vi "Generate Blend Points.vi"(6 "Index":i32, 8 "Speeds":T2={"maxV (fps)"=20.0, "Accel Limit (fps^2)"=20.0, "Initial V (fps)"=0.0, "Sample Period (s)"=0.02, "Jerk Limit (fps^3)"=0.0, "Jerk Distances"={"distance (ft)"=0.0, 0.0, 0.0}, "Jerk Distances"={"distance (ft)"=0.0, 0.0, 0.0}}, 9 "Initial Point":cluster{"x":dbl, "y":dbl, "th":dbl}={"x"=1.0, "y"=2.0, "th"=30.0}, 10 "Initial Acceleration":dbl format="%#_13g", 11 "Blend Info":T1) -> (0 "Speeds Out":T2={"maxV (fps)"=20.0, "Accel Limit (fps^2)"=20.0, "Initial V (fps)"=0.0, "Sample Period (s)"=0.02, "Jerk Limit (fps^3)"=0.0, "Jerk Distances"={"distance (ft)"=0.0, 0.0, 0.0}, "Jerk Distances"={"distance (ft)"=0.0, 0.0, 0.0}}, 3 "Trajectory Segment":T3, 5 "Final Acceleration":dbl)   [LabVIEW 2019]
uses:
  BlendType.ctl
panel:
  out "XY Graph":cluster{cluster{dbl, dbl}[]}[](graph)
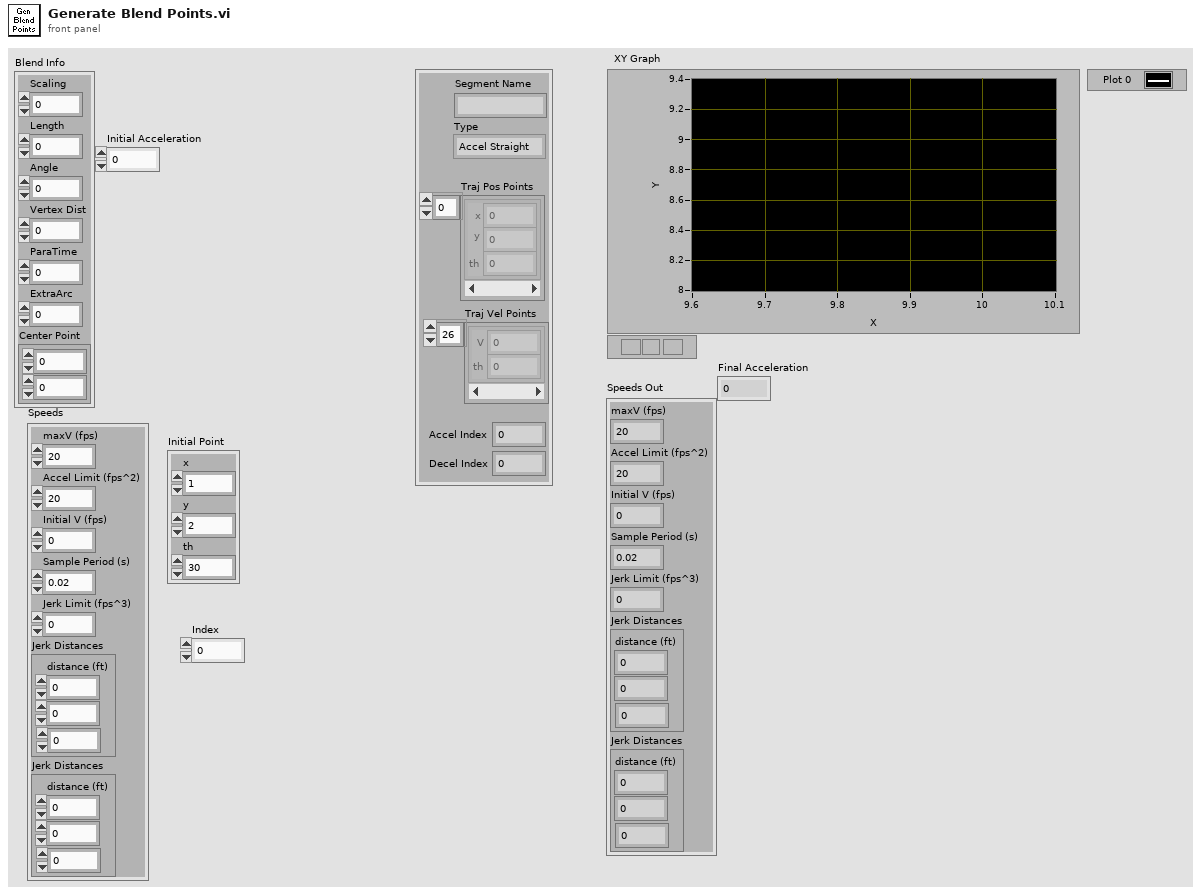
[diagram p1: front panel]
types:
  T1 = typedef "BlendType.ctl" = cluster{"Scaling":dbl, "Length":dbl, "Angle":dbl, "Vertex Dist":dbl, "ParaTime":dbl, "ExtraArc":dbl, "Center Point":cluster{dbl, dbl}}
  T2 = cluster{"maxV (fps)":dbl, "Accel Limit (fps^2)":dbl, "Initial V (fps)":dbl, "Sample Period (s)":dbl, "Jerk Limit (fps^3)":dbl, "Jerk Distances":cluster{"distance (ft)":dbl, dbl, dbl}, "Jerk Distances":cluster{"distance (ft)":dbl, dbl, dbl}}
  T3 = cluster{"Segment Name":string, "Type":enum16{"Accel Straight", "Const Straight", "Blend", "Circle"}, "Traj Pos Points":cluster{"x":dbl, "y":dbl, "th":dbl}[], "Traj Vel Points":cluster{"V":dbl, "th":dbl}[], "Accel Index":i32, "Decel Index":i32}
  T4 = enum16{"Accel Straight", "Const Straight", "Blend", "Circle"}
  T5 = cluster{string, "Type":enum16{"Accel Straight", "Const Straight", "Blend", "Circle"}, cluster{dbl, dbl, dbl}[], cluster{dbl, dbl}[], "Accel Index":i32, "Decel Index":i32}
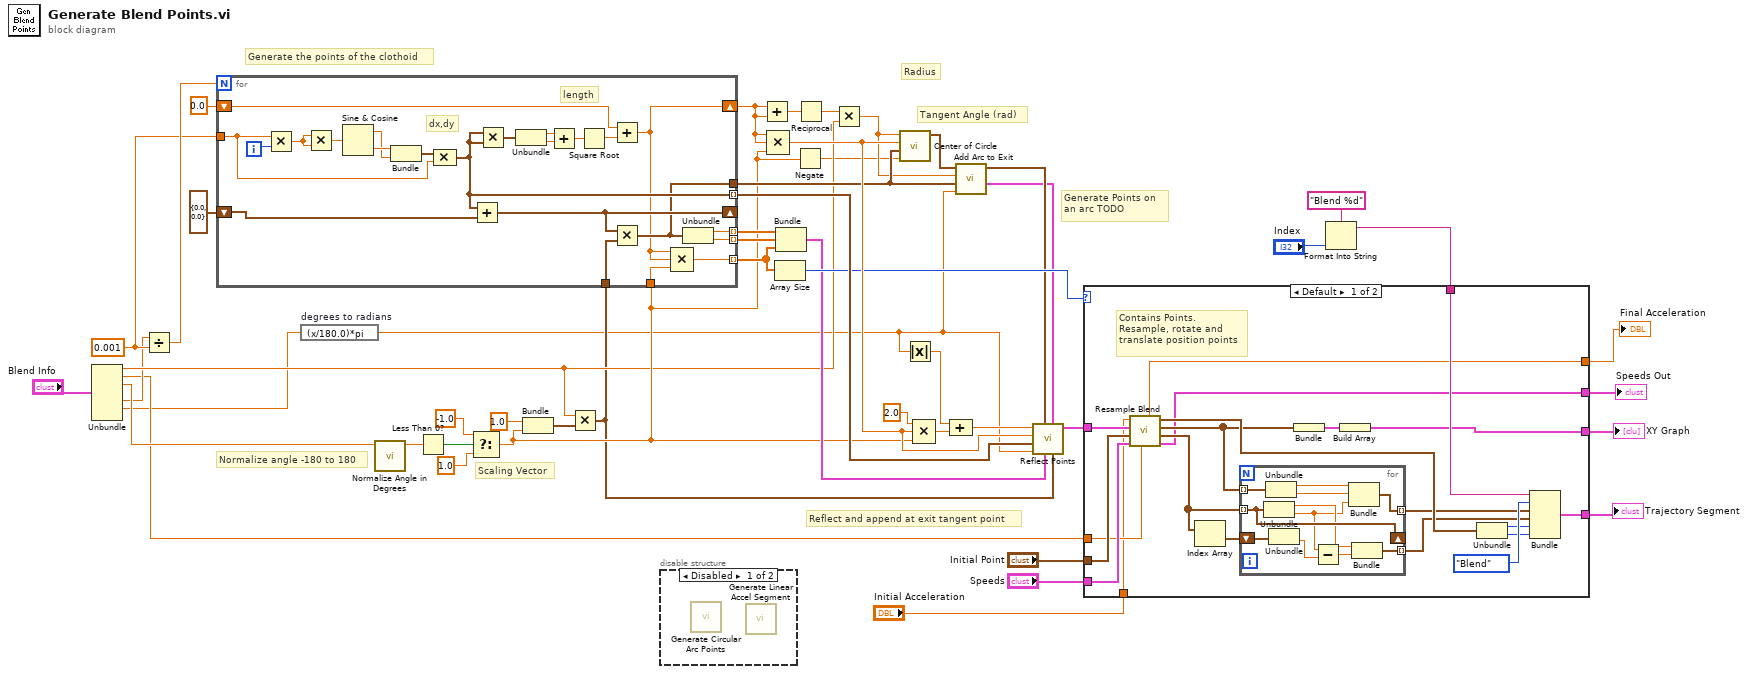
[diagram p0: block diagram]
diagram:
  w17 = 0.001
  # "Generate Points on \nan arc TODO"
  # "Reflect and append at exit tangent point"
  # "Scaling Vector"
  # "Normalize angle -180 to 180"
  # "Radius"
  # "Tangent Angle (rad)"
  # "Generate the points of the clothoid"
  n1 = Unbundle("Blend Info") -> ("Scaling"=w15:dbl, "Length"=w12:dbl, "Angle"=w14:dbl, "ParaTime"=w13:dbl, "ExtraArc"=w7:dbl)  [unwired: 2 out]
  n2 = Divide(x=w13, y=w17) -> (x/y=w49:dbl)
  n3 = expression code="(x/180.0)*pi" "degrees to radians"(w7) -> (w3:dbl)
  n4 = call "Normalize Angle in Degrees.vi"("Angle deg"=w14) -> ("Angle"=w28:dbl)  [unwired: 10 in]
  n5 = Less Than 0?(x=w28) -> (x < 0?=w31:bool)
  n6 = Select(t=-1.0, s=w31, f=1.0) -> (s? t:f=w22:dbl)
  n7 = Bundle(1.0, w22) -> (w29:cluster{dbl, dbl})  [unwired: 1 in]
  n8 = Multiply(x=w15, y=w29) -> (x*y=w5:cluster{dbl, dbl})
  n9 = for {
    N: w49 -> [_]
    shift-right: [w66] -> _
    shift-left: cluster{dbl, dbl} {0.0, 0.0} -> [w68]
    tunnel: w17 -> [w65]
    shift-right: [w55] -> w47
    shift-left: 0.0 -> [w60]
    tunnel: [w56] -> w42
    tunnel: [w58] -> w48 mode=indexing
    tunnel: w5 -> [w57]
    tunnel: [w52] -> w26 mode=indexing
    tunnel: [w51] -> w27 mode=indexing
    tunnel: w22 -> [w54]
    tunnel: [w53] -> w24 mode=indexing
    i -> [w73]
    # "length"
    # "dx,dy"
    n10 = Multiply(x=w65, y=w73) -> (x*y=w67:dbl)
    n11 = Multiply(x=w67, y=w67) -> (x*y=w72:dbl)
    n12 = Sine & Cosine(0:w72) -> (1:w70:dbl, 2:w71:dbl)
    n13 = Bundle(w71, w70) -> (w69:cluster{dbl, dbl})  [unwired: 1 in]
    n14 = Compound Arithmetic op=MULTIPLY(w69, w65) -> (w58:cluster{dbl, dbl})
    n15 = Add(x=w58, y=w68) -> (x+y=w66:cluster{dbl, dbl})
    n16 = Multiply(x=w58, y=w58) -> (x*y=w64:cluster{dbl, dbl})
    n17 = Unbundle(w64) -> (w63:dbl, w62:dbl)
    n18 = Add(x=w63, y=w62) -> (x+y=w61:dbl)
    n19 = Square Root(x=w61) -> (sqrt(x)=w59:dbl)
    n20 = Add(x=w60, y=w59) -> (x+y=w55:dbl)
    n21 = Multiply(x=w66, y=w57) -> (x*y=w56:cluster{dbl, dbl})
    n22 = Compound Arithmetic op=MULTIPLY(w55, w55, w54) -> (w53:dbl)
    n23 = Unbundle(w56) -> (w52:dbl, w51:dbl)
  }
  n24 = disable-structure shown="Disabled" {
    frame Disabled {
      n25 = call "Generate Circular Arc Points.vi"() -> ()  [unwired: 9 in, 3 out]
      n26 = call "Generate Linear Accel Segment.vi"() -> ()  [unwired: 7 in, 5 out]
    }
    frame Enabled {
    }
  }
  n27 = Add(x=w47, y=w47) -> (x+y=w46:dbl)
  n28 = Compound Arithmetic op=MULTIPLY(w47, w47, w22) -> (w44:dbl)
  n29 = Array Size(array=w24) -> (size(s)=w35:i32)
  n30 = Bundle(w26, w27, w24) -> (w25:cluster{dbl[], dbl[], dbl[]})  [unwired: 1 in]
  n31 = Negate(x=w22) -> (-x=w8:dbl)
  n32 = Reciprocal(x=w46) -> (1/x=w45:dbl)
  n33 = Multiply(x=w45, y=w15) -> (x*y=w41:dbl)
  n34 = call "Center of Circle.vi"("Sign"=w8, "Tangent Point"=w42, "Tangent Angle"=w44, "Radius"=w41) -> ("Center Point"=w43:cluster{dbl, dbl})  [unwired: 7 in]
  n35 = Absolute Value(x=w3) -> (abs(x)=w6:dbl)
  n36 = Compound Arithmetic op=MULTIPLY(2.0, w44, w22) -> (w18:dbl)
  n37 = Compound Arithmetic op=ADD(w6, w18) -> (w19:dbl)
  n38 = call "Add Arc to Exit.vi"("Additional circle arc (rad)"=w3, "Tangent Point"=w42, "Radius"=w41, "Center Point"=w43) -> ("Point Arrays"=w4:cluster{dbl[], dbl[], dbl[]}, "Blend Exit Point"=w21:cluster{dbl, dbl})  [unwired: 6 in]
  n39 = call "Reflect Points.vi"("Scaling Vector"=w5, "Arc Point Arrays"=w4, "Blend Point Arrays"=w25, "Blend Exit Point"=w21, "Extra Arc rad"=w3, "Delta Points"=w48, "Tangent Angle (rad)"=w44, "Angle"=w19) -> ("Point Arrays"=w23:cluster{dbl[], dbl[], dbl[]})  [unwired: 3 in]
  n40 = Format Into String(format string="Blend %d", "Index") -> (resulting string=w11:string)  [unwired: 2 in, 1 out]
  n41 = case shown="Default" w35 {
    tunnel: "Initial Point" -> [w89 _]
    tunnel: [w92 _] -> w38
    tunnel: "Speeds" -> [w87 w105]
    tunnel: w11 -> [w91 _]
    tunnel: [w90 _] -> w36
    tunnel: [w77 w105] -> w34
    tunnel: w23 -> [w76 _]
    tunnel: w12 -> [w86 _]
    tunnel: "Initial Acceleration" -> [w75 _]
    tunnel: [w74 _] -> w1
    frame Default {
      # "Contains Points.\nResample, rotate and\ntranslate position points"
      n42 = call "Resample Blend.vi"("Length"=w86, "Speeds"=w87, "Initial Point"=w89, "Point Arrays"=w76, "Initial Acceleration"=w75) -> ("Speeds Out"=w77:T2, "Vel Points"=w78:cluster{dbl, dbl}[], "Points"=w79:cluster{dbl, dbl}[], "Indices"=w85:cluster{"Accel Index":i32, "Decel Index":i32}, "Final Acceleration"=w74:dbl)  [unwired: 2 in]
      n43 = Index Array(array=w78) -> (element=w82:cluster{dbl, dbl})  [unwired: 1 in]
      n44 = for {
        tunnel: w79 -> [w104] mode=indexing
        tunnel: [w101] -> w80 mode=indexing
        tunnel: w78 -> [w97] mode=indexing
        shift-right: [w97] -> _
        shift-left: w82 -> [w99]
        tunnel: [w94] -> w81 mode=indexing
        n45 = Unbundle(w97) -> (w96:dbl, w95:dbl)
        n46 = Unbundle(w104) -> (w103:dbl, w102:dbl)
        n47 = Unbundle(w99) -> (w100:dbl)  [unwired: 1 out]
        n48 = Subtract(x=w95, y=w100) -> (x-y=w98:dbl)
        n49 = Bundle(w103, w102, w95) -> (w101:cluster{dbl, dbl, dbl})  [unwired: 1 in]
        n50 = Bundle(w96, w98) -> (w94:cluster{dbl, dbl})  [unwired: 1 in]
      }
      n51 = Bundle("Points"=w79) -> (w93:cluster{"Points":cluster{dbl, dbl}[]})  [unwired: 1 in]
      n52 = Build Array(w93) -> (w90:cluster{"Points":cluster{dbl, dbl}[]}[])
      n53 = Unbundle(w85) -> ("Accel Index"=w84:i32, "Decel Index"=w83:i32)
      n54 = Bundle(w91, "Type"=T4."Blend", w80, w81, "Accel Index"=w84, "Decel Index"=w83) -> (w92:T5)  [unwired: 1 in]
    }
    frame 0 {
    }
  }
  "Trajectory Segment" <- w38
  "XY Graph" <- w36
  "Speeds Out" <- w34
  "Final Acceleration" <- w1
